vi "trajCorrection.vi"(8 "goal Width":i32, 9 "goal X":dbl, 10 "BallRef":refnum<class "Ball.lvclass">) -> (2 "x":dbl, 3 "y":dbl)   [LabVIEW 2024, in "DefendGoalTactic.lvclass"]
uses:
  DefendGoalTactic.lvclass
  Ball_class/Ball.lvclass
  C:/Users/ROBOIME2/Documents/SSL ROBOIME/SSL_AI/Object_class/Object.lvclass
  Object_class/Object.lvclass/Object.ctl
  Ball_class/Ball.lvclass/Ball.ctl
  Object_class/Read x.vi
  Object_class/Read y.vi
  Ball_class/Read v_x.vi
  Ball_class/Read v_y.vi
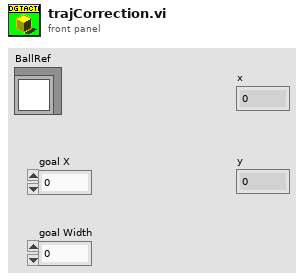
[diagram p1: front panel]
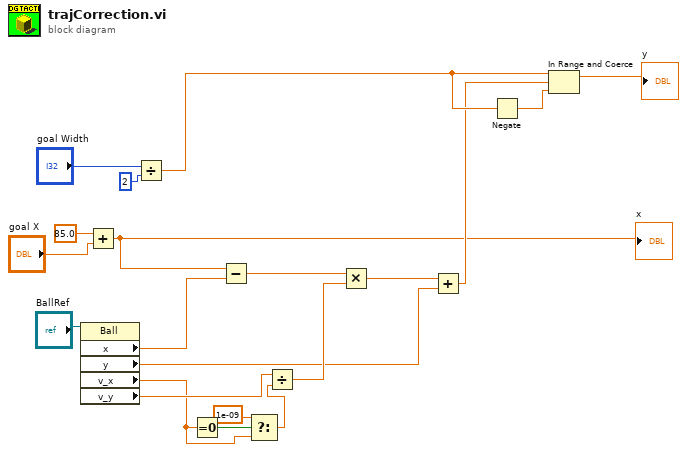
[diagram p0: block diagram]
diagram:
  n1 = property class="Ball"(reference="BallRef") -> ("x"=w14:dbl, "y"=w9:dbl, "v_x"=w1:dbl, "v_y"=w13:dbl)  [unwired: 1 in, 2 out]
  n2 = Add(x=85.0, y="goal X") -> (x+y=w7:dbl)
  "x" <- w7
  n3 = Divide(x="goal Width", y=2) -> (x/y=w16:dbl)
  n4 = Equal To 0?(x=w1) -> (x = 0?=w4:bool)
  n5 = Subtract(x=w7, y=w14) -> (x-y=w12:dbl)
  n6 = Select(t=1e-09, s=w4, f=w1) -> (s? t:f=w2:dbl)
  n7 = Divide(x=w13, y=w2) -> (x/y=w11:dbl)
  n8 = Multiply(x=w12, y=w11) -> (x*y=w10:dbl)
  n9 = Add(x=w10, y=w9) -> (x+y=w8:dbl)
  n10 = Negate(x=w16) -> (-x=w15:dbl)
  n11 = In Range and Coerce(upper limit=w16, x=w8, lower limit=w15) -> (coerced(x)=→"y":dbl)  [unwired: 1 out]
